vi "New (Element).vi"(8 "error in (no error)":errorcluster, 10 "match behavior (keep)":T1, 11 "regex string":string) -> (0 "error out":errorcluster, 3 "regex out":refnum<class "Regex.lvclass">)   [LabVIEW 2024, in "Logging.lvlib" / "Regex.lvclass"]
uses:
  Regex.lvclass
  Regex.lvclass/Regex.ctl
  <vilib>/regexp/Match Regular Expression.xnode
  Aggregation Method.ctl
  Logging.lvlib
  Filter/Filter.lvclass
  Match Behavior.ctl
panel:
  # "Connector Pane"
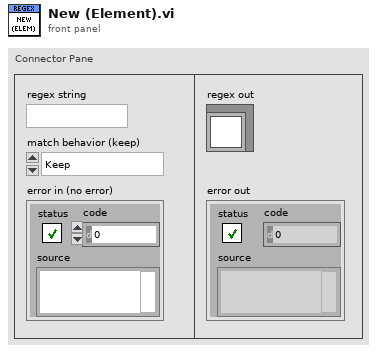
[diagram p1: front panel]
types:
  T1 = typedef "Logging.lvlib/Match Behavior.ctl" = enum16{"Keep", "Discard"}
  T2 = typedef "Logging.lvlib/Aggregation Method.ctl" = enum16{"Any", "Only", "All", "None"}
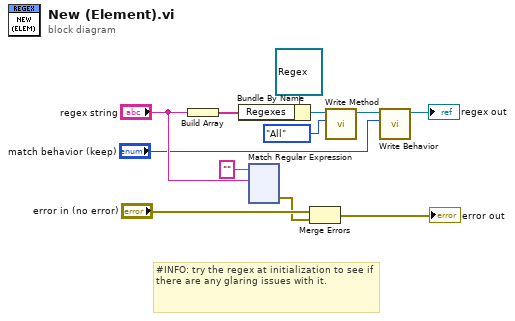
[diagram p0: block diagram]
diagram:
  # "#INFO: try the regex at initialization to see if there are any glaring issues with it."
  n1 = Build Array("regex string") -> (w5:string[])
  n2 = Bundle By Name(cluster=refnum<class "Regex.lvclass"> refnum ("Regex in"), "Regexes"=w5) -> (w11:refnum<class "Regex.lvclass">)
  n3 = xnode "Match Regular Expression"("input string"="", "regular expression"="regex string") -> ("error out"=w8:errorcluster)  [unwired: 4 in, 4 out]
  n4 = Merge Errors("error in (no error)", w8) -> (→"error out":errorcluster)
  n5 = call "Write Method.vi"("Method"=Aggregation_Method."All", "Filter in"=w11) -> ("Filter out"=w4:refnum<class "Regex.lvclass">)  [unwired: 9 in]
  n6 = call "Write Behavior.vi"("match behavior"="match behavior (keep)", "Filter in"=w4) -> ("Filter out"=→"regex out":refnum<class "Regex.lvclass">)  [unwired: 9 in]
